vi "Inovance_Set_Trigger_Mode_SubVI.vi"(8 "error in (no error)":errorcluster, 10 "Trigger Mode":enum16{"Free Run", "Hardware"}(ring), 11 "Refnum in":T1) -> (0 "error out":errorcluster, 3 "Refnum out":T1)   [LabVIEW 2023, in "Inovance_Camera.lvlib"]
uses:
  Inovance_Camera.lvlib
  <vilib>/userDefined/High Color/IMAQdx.ctl
  <resource>/objmgr/imaqdx.rc
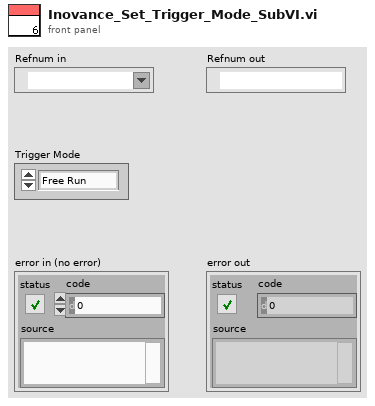
[diagram p1: front panel]
types:
  T1 = typedef "IMAQdx.ctl" = refnum<k21>
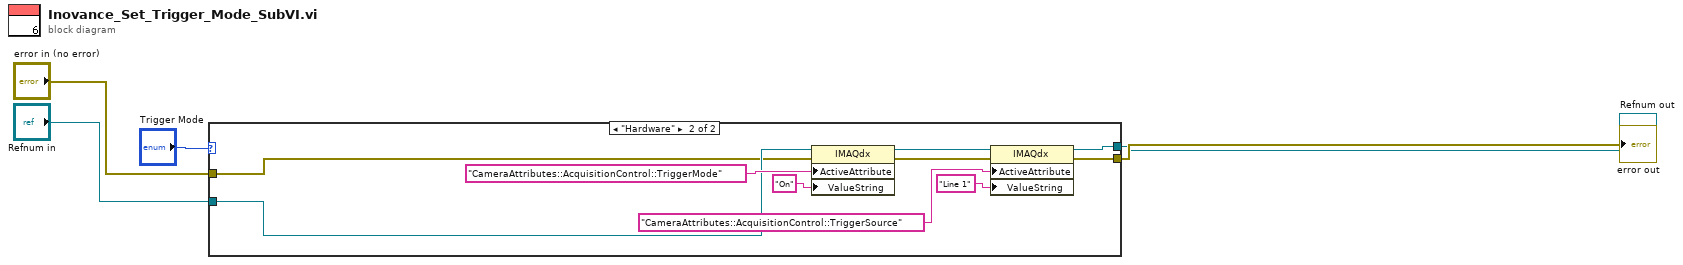
[diagram p0: block diagram]
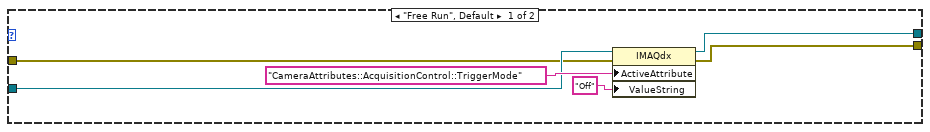
[diagram p2: hidden frame]
diagram:
  n1 = case shown="\"Hardware\"" "Trigger Mode" {
    tunnel: "Refnum in" -> [w10 w20]
    tunnel: [w9 w15] -> w2
    tunnel: "error in (no error)" -> [w6 w13]
    tunnel: [w7 w12] -> w4
    frame "Free Run", Default {
      n2 = property class="IMAQdx"(reference=w10, error in=w6, "ActiveAttribute"="CameraAttributes::AcquisitionControl::TriggerMode", "ValueString"="Off") -> (reference out=w9:T1, error out=w7:errorcluster)
    }
    frame "Hardware" {
      n3 = property class="IMAQdx"(reference=w20, error in=w13, "ActiveAttribute"="CameraAttributes::AcquisitionControl::TriggerMode", "ValueString"="On") -> (reference out=w16:T1, error out=w14:errorcluster)
      n4 = property class="IMAQdx"(reference=w16, error in=w14, "ActiveAttribute"="CameraAttributes::AcquisitionControl::TriggerSource", "ValueString"="Line 1") -> (reference out=w15:T1, error out=w12:errorcluster)
    }
  }
  "error out" <- w4
  "Refnum out" <- w2
